vi "TTL Continuous Output.vi"() -> ()   [LabVIEW 2012]
uses:
  <vilib>/DAQmx/create/channels.llb/DAQmx Create Channel (DO-Digital Output).vi
  <vilib>/DAQmx/write.llb/DAQmx Write (Digital Bool 1Line 1Point).vi
panel:
  out ".not. x?":bool
  in  "stop":bool
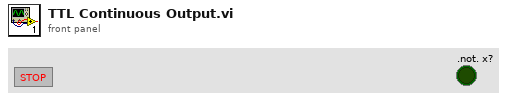
[diagram p1: front panel]
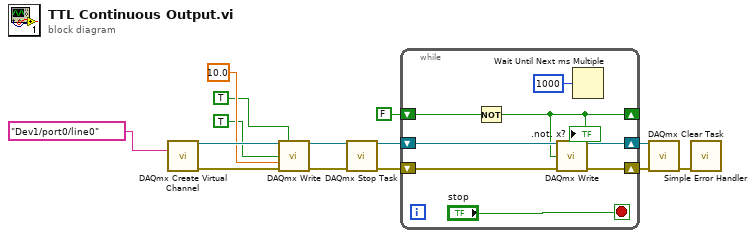
[diagram p0: block diagram]
diagram:
  n1 = call-poly <vilib>:"DAQmx Create Virtual Channel.vi"("lines"=tag "Dev1/port0/line0") -> ("task out"=w12:refnum<k21>, "error out"=w13:errorcluster)  [unwired: 13 in]
  n2 = call-poly <vilib>:"DAQmx Write.vi"("task/channels in"=w12, "auto start"=TRUE, "data"=TRUE, "timeout"=10.0, "error in"=w13) -> ("task out"=w7:refnum<k21>, "error out"=w11:errorcluster)  [unwired: 8 in, 1 out]
  n3 = call <vilib>:"DAQmx Stop Task.vi"("task/channels in"=w7, "error in"=w11) -> ("task out"=w6:refnum<k21>, "error out"=w8:errorcluster)  [unwired: 12 in]
  n4 = while {
    shift-right: [w19] -> w4
    shift-left: w8 -> [w22]
    shift-right: [w20] -> w5
    shift-left: w6 -> [w21]
    shift-right: [w15] -> _
    shift-left: FALSE -> [w16]
    stop <- "stop" stop-if-true
    n5 = Not(x=w16) -> (.not. x?=w15:bool)
    ".not. x?" <- w15
    n6 = call-poly <vilib>:"DAQmx Write.vi"("task/channels in"=w21, "data"=w15, "error in"=w22) -> ("task out"=w20:refnum<k21>, "error out"=w19:errorcluster)  [unwired: 10 in, 1 out]
    n7 = Wait Until Next ms Multiple(millisecond multiple=u32 1000) -> ()  [unwired: 1 out]
  }
  n8 = call <vilib>:"DAQmx Clear Task.vi"("task in"=w5, "error in"=w4) -> ("error out"=w3:errorcluster)  [unwired: 13 in]
  n9 = call <vilib>:"Simple Error Handler.vi"("error in (no error)"=w3) -> ()  [unwired: 4 in, 5 out]
